vi "get depth frame.vi"(8 "error in (no error)":errorcluster, 10 "fmt":T1(ring), 11 "index":i32) -> (0 "error out":errorcluster, 3 "Destination":u16[](array[numeric]))   [LabVIEW 2017, in "libfreenect.lvlib"]
doc: "EXPORT short *freenect_lv_get_depth_frame(int index, freenect_depth_format fmt);"
uses:
  libfreenect.lvlib
  freenect_lv.dll
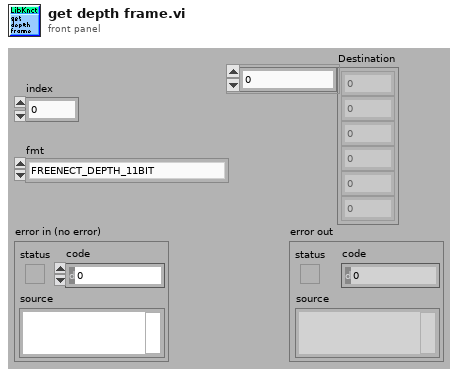
[diagram p1: front panel]
types:
  T1 = enum16{"FREENECT_DEPTH_11BIT", "FREENECT_DEPTH_10BIT", "FREENECT_DEPTH_11BIT_PACKED", "FREENECT_DEPTH_10BIT_PACKED"}
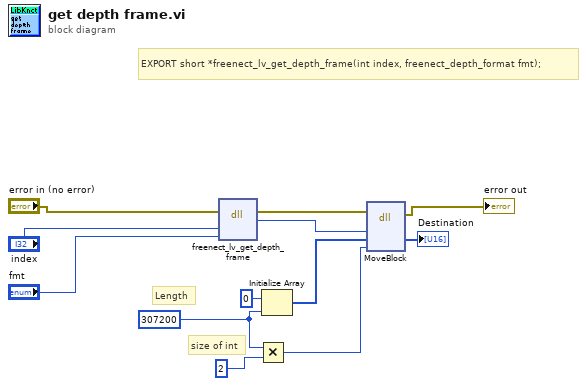
[diagram p0: block diagram]
diagram:
  w4 = 307200 ("dimension size")
  # "size of int"
  # "Length"
  # "EXPORT short *freenect_lv_get_depth_frame(int index, freenect_depth_format fmt);"
  n1 = dll-call lib="C:/Users/Mats/Desktop/Bacheler prosjekt/Labview/Occupancy Grid Map Code - With model/freenect_lv.*" fn="freenect_lv_get_depth_frame"(error in="error in (no error)", "index"="index", "fmt"="fmt") -> (error out=w7:errorcluster, "return type"=w8:i64)  [unwired: 3 in, 2 out]
  n2 = Multiply(x=w4, y=2) -> (x*y=w2:i32)
  n3 = Initialize Array(u16 0 ("element"), w4) -> (w5:u16[])
  n4 = dll-call lib="LabVIEW" fn="MoveBlock"(error in=w7, "Address (Pointer)"=w8, "Destination"=w5, "Size"=w2) -> (error out=→"error out":errorcluster, "Destination"=→"Destination":u16[])  [unwired: 4 in, 2 out]
